vi "Create Engine Source Distribution.vi"(6 "Base Path":path, 8 "error in (no error)":errorcluster, 9 "Library Refnum":refnum<vi>, 10 "Project Refnum":refnum<vi>, 11 "Custom Device Name":string) -> (0 "error out":errorcluster)   [LabVIEW 2020, in "Custom Device Template Tool.lvlib"]
uses:
  <vilib>/NI VeriStand/Custom Device Tools/Custom Device Template Tool/Custom Device Template Tool.lvlib
  <vilib>/AppBuilder/AB_API/common/AB_API Default Destinations.ctl
  <vilib>/AppBuilder/AB_API/common/AB_API Path Exclusions.ctl
  <vilib>/AppBuilder/AB_API/common/AB_API Primary Exclusions.ctl
  <vilib>/AppBuilder/AB_API/common/AB_API Destination Type.ctl
  <vilib>/AppBuilder/AB_API/SDIST/NI_AB_API_SDIST.lvclass
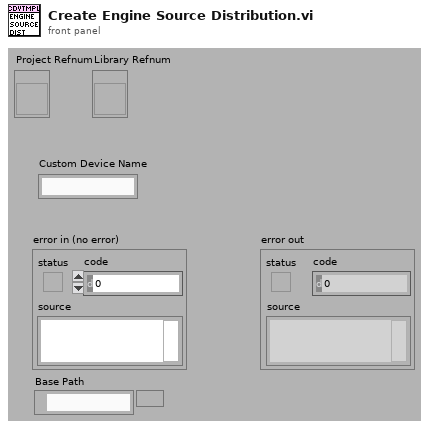
[diagram p1: front panel]
types:
  T1 = typedef "AB_API Default Destinations.ctl" = enum16{"Destination Directory", "Support Directory"}
  T2 = typedef "AB_API Path Exclusions.ctl" = cluster{"Exclude files from vi.lib":bool, "Exclude files from instr.lib":bool, "Exclude files from user.lib":bool}
  T3 = typedef "AB_API Primary Exclusions.ctl" = cluster{"Disconnect type definitions":bool, "Remove unused polymorphic VI instances":bool, "Remove unused members of project libraries":bool, "Modify project library file after removing unused members":bool}
  T4 = typedef "AB_API Destination Type.ctl" = enum16{"directory", "directory (preserve hierarchy)", "LLB"}
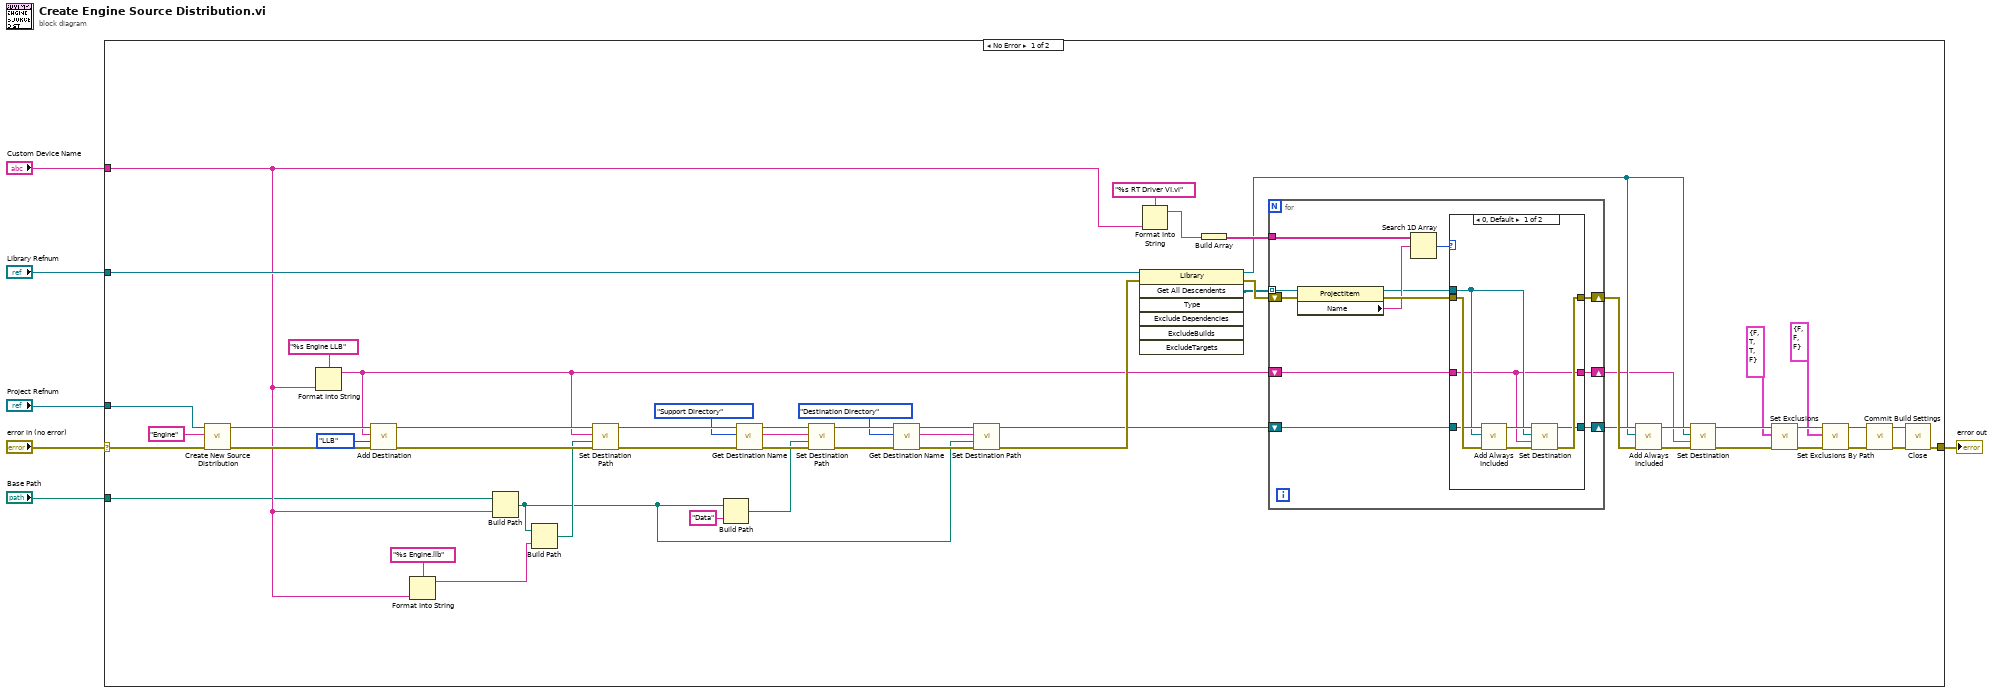
[diagram p0: block diagram]
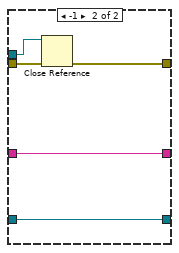
[diagram p2: hidden frame]
diagram:
  n1 = case shown="No Error" "error in (no error)" {
    selector: "error in (no error)" -> [w54 w87]
    tunnel: [w32 w87] -> w6
    tunnel: "Project Refnum" -> [w53 _]
    tunnel: "Library Refnum" -> [w51 _]
    tunnel: "Custom Device Name" -> [w40 _]
    tunnel: "Base Path" -> [w21 _]
    frame No Error {
      n2 = call <vilib>:"Create New Source Distribution.vi"("error in (no error)"=w54, "Build specification name"="Engine", "Project Refnum"=w53) -> ("error out"=w44:errorcluster, "SDIST out"=w57:refnum<class "NI_AB_API_SDIST.lvclass">)  [unwired: 7 in]
      n3 = Format Into String(format string="%s Engine LLB", w40) -> (resulting string=w39:string)  [unwired: 2 in, 1 out]
      n4 = call-dynamic "Add Destination.vi"("error in (no error)"=w44, "Destination type (directory)"=AB_API_Destination_Type."LLB", "Destination label"=w39, "SDIST in"=w57) -> ("error out"=w22:errorcluster, "SDIST out"=w46:refnum<class "NI_AB_API_SDIST.lvclass">)  [unwired: 6 in]
      n5 = Format Into String(format string="%s Engine.llb", w40) -> (resulting string=w41:string)  [unwired: 2 in, 1 out]
      n6 = Build Path(base path=w21, name or relative path=w40) -> (appended path=w17:path)
      n7 = Build Path(base path=w17, name or relative path=w41) -> (appended path=w20:path)
      n8 = call-dynamic "Set Destination Path.vi"("error in (no error)"=w22, "Destination path"=w20, "Destination label"=w39, "SDIST in"=w46) -> ("error out"=w14:errorcluster, "SDIST out"=w15:refnum<class "NI_AB_API_SDIST.lvclass">)  [unwired: 6 in]
      n9 = Build Path(base path=w17, name or relative path="Data") -> (appended path=w18:path)
      n10 = call-dynamic "Get Destination Name.vi"("error in (no error)"=w14, "Default Destinations"=AB_API_Default_Destinations."Support Directory", "SDIST in"=w15) -> ("error out"=w59:errorcluster, "Destination Name"=w7:string, "SDIST out"=w13:refnum<class "NI_AB_API_SDIST.lvclass">)  [unwired: 6 in]
      n11 = call-dynamic "Set Destination Path.vi"("error in (no error)"=w59, "Destination path"=w18, "Destination label"=w7, "SDIST in"=w13) -> ("error out"=w10:errorcluster, "SDIST out"=w61:refnum<class "NI_AB_API_SDIST.lvclass">)  [unwired: 6 in]
      n12 = call-dynamic "Get Destination Name.vi"("error in (no error)"=w10, "Default Destinations"=AB_API_Default_Destinations."Destination Directory", "SDIST in"=w61) -> ("error out"=w60:errorcluster, "Destination Name"=w8:string, "SDIST out"=w9:refnum<class "NI_AB_API_SDIST.lvclass">)  [unwired: 6 in]
      n13 = call-dynamic "Set Destination Path.vi"("error in (no error)"=w60, "Destination path"=w17, "Destination label"=w8, "SDIST in"=w9) -> ("error out"=w58:errorcluster, "SDIST out"=w16:refnum<class "NI_AB_API_SDIST.lvclass">)  [unwired: 6 in]
      n14 = invoke class="Library" method="Get All Descendents"(reference=w51, error in=w58) -> (reference out=w36:refnum<vi>, error out=w55:errorcluster, "All Descendents"=w50:refnum<vi>[])  [unwired: 5 in, 4 out]
      n15 = Format Into String(format string="%s RT Driver VI.vi", w40) -> (resulting string=w49:string)  [unwired: 2 in, 1 out]
      n16 = Build Array(w49) -> (w48:string[])
      n17 = for {
        tunnel: w50 -> [w72] mode=indexing
        shift-right: [w66] -> w56
        shift-left: w55 -> [w71]
        tunnel: w48 -> [w70]
        shift-right: [w64] -> w47
        shift-left: w16 -> [w65]
        shift-right: [w62] -> w35
        shift-left: w39 -> [w63]
        n18 = property class="ProjectItem"(reference=w72, error in=w71) -> (reference out=w67:refnum<vi>, error out=w73:errorcluster, "Name"=w69:string)
        n19 = Search 1D Array(1D array=w70, element=w69) -> (index of element=w68:i32)  [unwired: 1 out]
        n20 = case shown="0, Default" w68 {
          tunnel: w73 -> [w81 w86]
          tunnel: w67 -> [w75 w85]
          tunnel: [w77 w84] -> w66
          tunnel: w65 -> [w80 w83]
          tunnel: [w76 w83] -> w64
          tunnel: w63 -> [w74 w82]
          tunnel: [w74 w82] -> w62
          frame 0, Default {
            n21 = call-dynamic "Add Always Included.vi"("error in (no error)"=w81, "ProjectItem Refnum"=w75, "SDIST in"=w80) -> ("error out"=w78:errorcluster, "SDIST out"=w79:refnum<class "NI_AB_API_SDIST.lvclass">)  [unwired: 7 in]
            n22 = call-dynamic "Set Destination.vi"("error in (no error)"=w78, "Destination label"=w74, "ProjectItem Refnum"=w75, "SDIST in"=w79) -> ("error out"=w77:errorcluster, "SDIST out"=w76:refnum<class "NI_AB_API_SDIST.lvclass">)  [unwired: 6 in]
          }
          frame -1 {
            n23 = Close Reference(reference=w85, error in (no error)=w86) -> (error out=w84:errorcluster)
          }
        }
      }
      n24 = call-dynamic "Add Always Included.vi"("error in (no error)"=w56, "ProjectItem Refnum"=w36, "SDIST in"=w47) -> ("error out"=w38:errorcluster, "SDIST out"=w37:refnum<class "NI_AB_API_SDIST.lvclass">)  [unwired: 7 in]
      n25 = call-dynamic "Set Destination.vi"("error in (no error)"=w38, "Destination label"=w35, "ProjectItem Refnum"=w36, "SDIST in"=w37) -> ("error out"=w30:errorcluster, "SDIST out"=w31:refnum<class "NI_AB_API_SDIST.lvclass">)  [unwired: 6 in]
      n26 = call-dynamic "Set Exclusions.vi"("error in (no error)"=w30, "Exclusions"=T3 {"Disconnect type definitions"=FALSE, "Remove unused polymorphic VI instances"=TRUE, "Remove unused members of project libraries"=TRUE, "Modify project library file after removing unused members"=FALSE}, "SDIST in"=w31) -> ("error out"=w27:errorcluster, "SDIST out"=w28:refnum<class "NI_AB_API_SDIST.lvclass">)  [unwired: 7 in]
      n27 = call-dynamic "Set Exclusions By Path.vi"("error in (no error)"=w27, "Path exclusions"=T2 {"Exclude files from vi.lib"=FALSE, "Exclude files from instr.lib"=FALSE, "Exclude files from user.lib"=FALSE}, "SDIST in"=w28) -> ("error out"=w25:errorcluster, "SDIST out"=w26:refnum<class "NI_AB_API_SDIST.lvclass">)  [unwired: 7 in]
      n28 = call-dynamic "Commit Build Settings.vi"("error in (no error)"=w25, "SDIST in"=w26) -> ("error out"=w33:errorcluster, "SDIST out"=w34:refnum<class "NI_AB_API_SDIST.lvclass">)  [unwired: 8 in]
      n29 = call-dynamic "Close.vi"("error in (no error)"=w33, "SDIST in"=w34) -> ("error out"=w32:errorcluster)  [unwired: 9 in]
    }
    frame Error {
    }
  }
  "error out" <- w6
